vi "Cage controller.vi"(5 "Action":T2, 7 "Set/Get":T1, 8 "error in (no error)":errorcluster, 9 "Cluster In":T3, 11 "reference in":refnum<k24>) -> (0 "error out":errorcluster, 1 "Cluster out":T3, 3 "reference out":refnum<k24>)   [LabVIEW 2018]
uses:
  Thorlabs Translation Stages/Controls/Translation Stage Cluster.ctl
  General/Controls/Translation Stage Types.ctl
  Thorlabs Translation Stages/Controls/Motion Translation Module Control.ctl
  General/Controls/Set Get Controls.ctl
  C:/Project/SerialSectionOCT/SerialSectOCT/Labview Software/Thorlabs.MotionControl.Controls.dll
  Thorlabs.MotionControl.Controls.dll
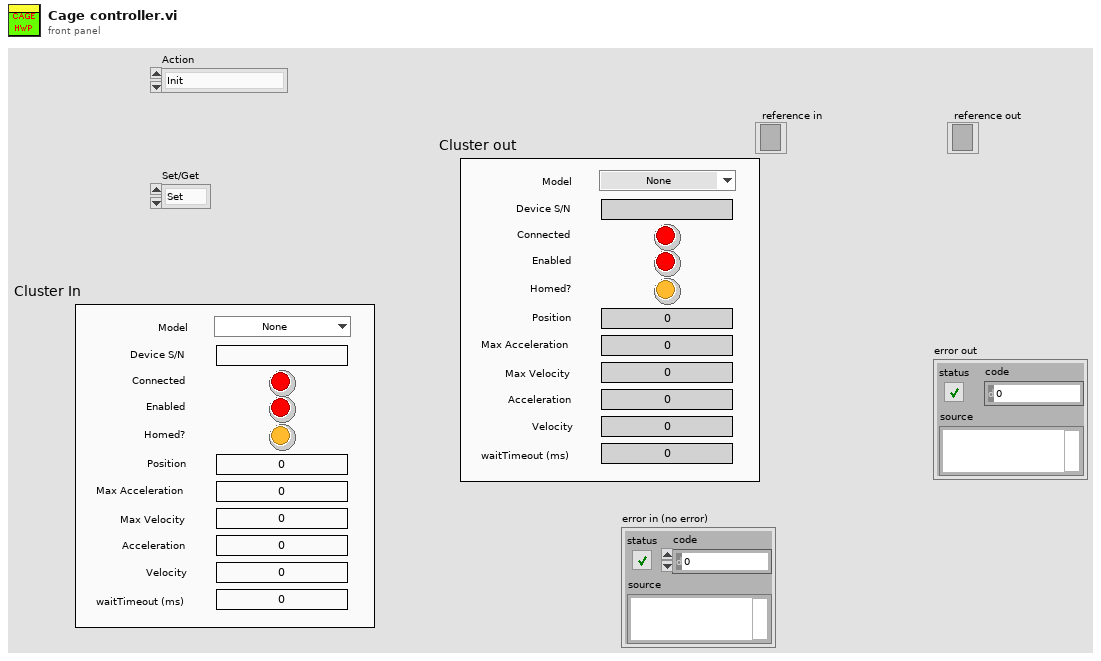
[diagram p1: front panel]
types:
  T1 = typedef "Set Get Controls.ctl" = enum16{"Set", "Get"}
  T2 = typedef "Motion Translation Module Control.ctl" = enum16{"Init", "Home", "Status", "Velocity/Accel", "Position", "Jog", "Stop", "Uninit", "Enable", "Disable"}
  T3 = typedef "Translation Stage Cluster.ctl" = cluster{"Position":dbl, "Is.Enabled?":bool, "Is.Connected?":bool, "Device SN":string, "AccelerationMaximum":dbl, "VelocityMaximum":dbl, "Acceleration":dbl, "Velocity":dbl, "waitTimeout (ms)":i32, "Model":T4, "Is.Homed?":bool}
  T4 = typedef "Translation Stage Types.ctl" = enum16{"None", "Thorlabs LTS", "Thorlabs MLJ"}
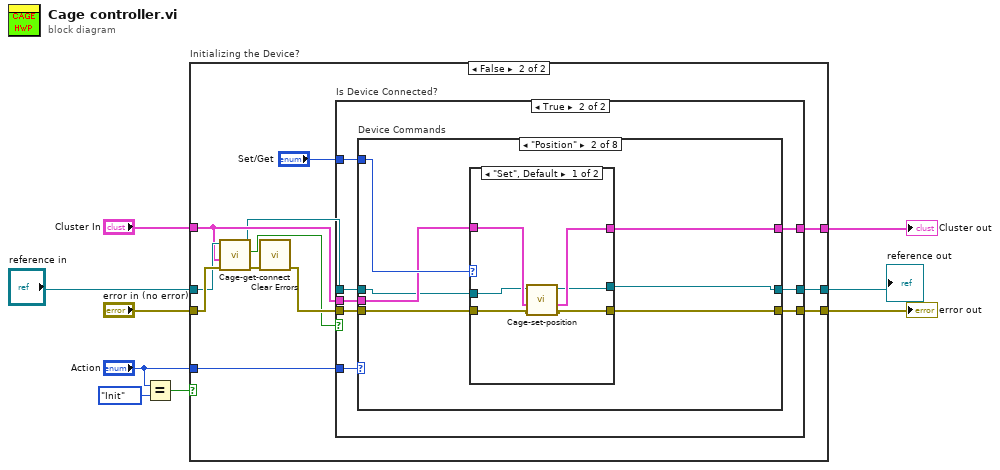
[diagram p0: block diagram]
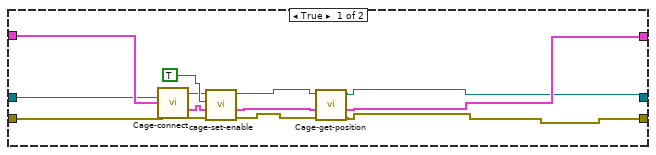
[diagram p2: hidden frame]
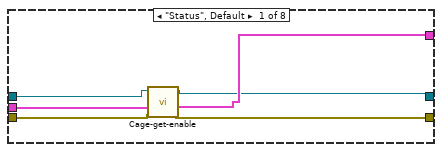
[diagram p4: hidden frame]
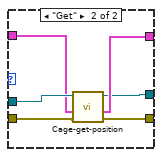
[diagram p5: hidden frame]
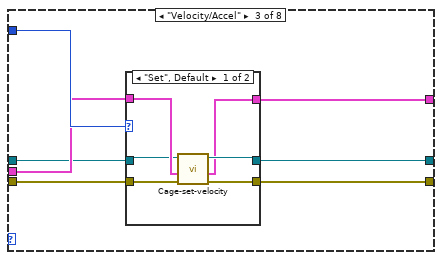
[diagram p6: hidden frame]
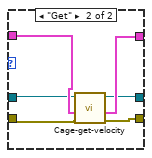
[diagram p7: hidden frame]
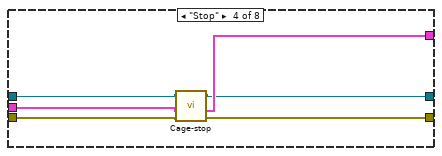
[diagram p8: hidden frame]
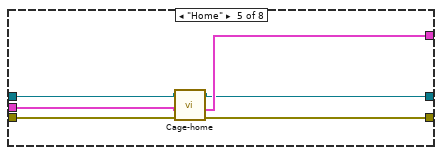
[diagram p9: hidden frame]
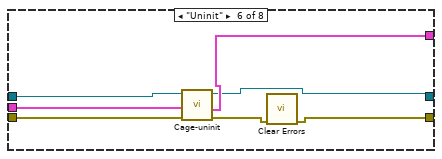
[diagram p10: hidden frame]
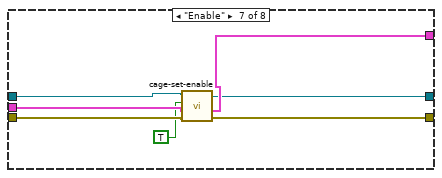
[diagram p11: hidden frame]
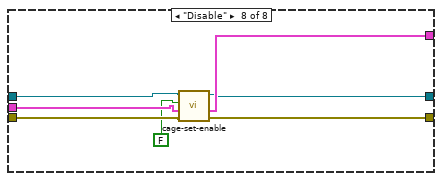
[diagram p12: hidden frame]
diagram:
  n1 = Equal?(x="Action", y=Motion_Translation_Module_Control."Init") -> (x = y?=w2:bool)
  n2 = case "Initializing the Device?" shown="False" w2 {
    tunnel: "reference in" -> [w20 w26]
    tunnel: [w10 w34] -> w9
    tunnel: [w11 w33] -> w8
    tunnel: [w12 w32] -> w7
    tunnel: "error in (no error)" -> [w22 w27]
    tunnel: "Cluster In" -> [w21 w24]
    tunnel: "Action" -> [_ w31]
    frame True {
      n3 = call "Cage-connect.vi"("error in (no error)"=w22, "Cluster in"=w21, "reference in"=w20) -> ("error out"=w19:errorcluster, "Cluster out"=w18:T3, "reference out"=w16:refnum<k24>)  [unwired: 5 in, 1 out]
      n4 = call "cage-set-enable.vi"("error in (no error)"=w19, "Cluster in"=w18, "Enable?"=TRUE, "reference in"=w16) -> ("error out"=w15:errorcluster, "Cluster out"=w14:T3, "reference out"=w13:refnum<k24>)  [unwired: 5 in]
      n5 = call "Cage-get-position.vi"("error in (no error)"=w15, "Cluster in"=w14, "reference in"=w13) -> ("error out"=w12:errorcluster, "Cluster out"=w11:T3, "reference out"=w10:refnum<k24>)  [unwired: 5 in, 1 out]
    }
    frame False {
      n6 = call "Cage-get-connect.vi"("error in (no error)"=w27, "Cluster in"=w24, "reference in"=w26) -> ("error out"=w28:errorcluster, "IsConnected"=w25:bool, "reference out"=w23:refnum<k24>)  [unwired: 5 in, 1 out]
      n7 = call <vilib>:"Clear Errors.vi"("error in (no error)"=w28) -> ("error out"=w29:errorcluster)  [unwired: 5 in, 1 out]
      n8 = case "Is Device Connected?" shown="True" w25 {
        tunnel: w23 -> [w35 w45]
        tunnel: [w35 w44] -> w34
        tunnel: [w37 w43] -> w33
        tunnel: [w36 w42] -> w32
        tunnel: w29 -> [w36 w41]
        tunnel: "Set/Get" -> [_ w40]
        tunnel: w31 -> [_ w39]
        tunnel: w24 -> [w37 w38]
        frame False {
        }
        frame True {
          n9 = case "Device Commands" shown="\"Position\"" w39 {
            tunnel: w40 -> [_ w58 w77 _ _ _ _ _]
            tunnel: w38 -> [w50 w55 w74 w94 w98 w106 w114 w121]
            tunnel: w41 -> [w51 w57 w76 w95 w101 w107 w115 w122]
            tunnel: [w47 w53 w72 w90 w96 w102 w109 w116] -> w44
            tunnel: [w46 w56 w75 w92 w100 w108 w111 w117] -> w42
            tunnel: [w48 w54 w73 w93 w99 w103 w110 w118] -> w43
            tunnel: w45 -> [w49 w52 w71 w91 w97 w105 w113 w120]
            frame "Status", Default {
              n10 = call "Cage-get-enable.vi"("error in (no error)"=w51, "Cluster in"=w50, "reference in"=w49) -> ("error out"=w46:errorcluster, "Cluster out"=w48:T3, "reference out"=w47:refnum<k24>)  [unwired: 5 in, 1 out]
            }
            frame "Position" {
              n11 = case shown="\"Set\", Default" w58 {
                tunnel: w57 -> [w64 w70]
                tunnel: [w63 w66] -> w56
                tunnel: w55 -> [w61 w68]
                tunnel: [w62 w67] -> w54
                tunnel: w52 -> [w60 w69]
                tunnel: [w59 w65] -> w53
                frame "Set", Default {
                  n12 = call "Cage-set-position.vi"("error in (no error)"=w64, "Cluster in"=w61, "reference in"=w60) -> ("error out"=w63:errorcluster, "Cluster out"=w62:T3, "reference out"=w59:refnum<k24>)  [unwired: 6 in]
                }
                frame "Get" {
                  n13 = call "Cage-get-position.vi"("error in (no error)"=w70, "Cluster in"=w68, "reference in"=w69) -> ("error out"=w66:errorcluster, "Cluster out"=w67:T3, "reference out"=w65:refnum<k24>)  [unwired: 5 in, 1 out]
                }
              }
            }
            frame "Velocity/Accel" {
              n14 = case shown="\"Set\", Default" w77 {
                tunnel: w76 -> [w83 w89]
                tunnel: [w82 w88] -> w75
                tunnel: w74 -> [w79 w87]
                tunnel: [w80 w86] -> w73
                tunnel: w71 -> [w78 w85]
                tunnel: [w81 w84] -> w72
                frame "Set", Default {
                  n15 = call "Cage-set-velocity.vi"("error in (no error)"=w83, "Cluster in"=w79, "reference in"=w78) -> ("error out"=w82:errorcluster, "Cluster out"=w80:T3, "reference out"=w81:refnum<k24>)  [unwired: 5 in, 1 out]
                }
                frame "Get" {
                  n16 = call "Cage-get-velocity.vi"("error in (no error)"=w89, "Cluster in"=w87, "reference in"=w85) -> ("error out"=w88:errorcluster, "Cluster out"=w86:T3, "reference out"=w84:refnum<k24>)  [unwired: 5 in, 1 out]
                }
              }
            }
            frame "Stop" {
              n17 = call "Cage-stop.vi"("error in (no error)"=w95, "Cluster in"=w94, "reference in"=w91) -> ("error out"=w92:errorcluster, "Cluster out"=w93:T3, "reference out"=w90:refnum<k24>)  [unwired: 6 in]
            }
            frame "Home" {
              n18 = call "Cage-home.vi"("error in (no error)"=w101, "Cluster in"=w98, "reference in"=w97) -> ("error out"=w100:errorcluster, "Cluster out"=w99:T3, "reference out"=w96:refnum<k24>)  [unwired: 6 in]
            }
            frame "Uninit" {
              n19 = call "Cage-uninit.vi"("error in (no error)"=w107, "Cluster in"=w106, "reference in"=w105) -> ("error out"=w104:errorcluster, "Cluster out"=w103:T3, "reference out"=w102:refnum<k24>)  [unwired: 5 in, 1 out]
              n20 = call <vilib>:"Clear Errors.vi"("error in (no error)"=w104) -> ("error out"=w108:errorcluster)  [unwired: 5 in, 1 out]
            }
            frame "Enable" {
              n21 = call "cage-set-enable.vi"("error in (no error)"=w115, "Cluster in"=w114, "Enable?"=TRUE, "reference in"=w113) -> ("error out"=w111:errorcluster, "Cluster out"=w110:T3, "reference out"=w109:refnum<k24>)  [unwired: 5 in]
            }
            frame "Disable" {
              n22 = call "cage-set-enable.vi"("error in (no error)"=w122, "Cluster in"=w121, "Enable?"=FALSE, "reference in"=w120) -> ("error out"=w117:errorcluster, "Cluster out"=w118:T3, "reference out"=w116:refnum<k24>)  [unwired: 5 in]
            }
          }
        }
      }
    }
  }
  "Cluster out" <- w8
  "error out" <- w7
  "reference out" <- w9
